vi "multi_column_list_box.vi"() -> ()   [LabVIEW 2023]
uses:
  Values.ctl
panel:
  out "error out":errorcluster
  in  "error in (no error)":errorcluster
  in  "Combo Box":T1
  in  "Multicolumn Listbox":i32[](listbox)=[4] caption="Table"
  in  "stop":bool
  # "Notes:\n    - Hovr the headers of the rows or column to highlisght the entire row or column.\n    - Select the valus present in the drop box to change the vale of the cell."
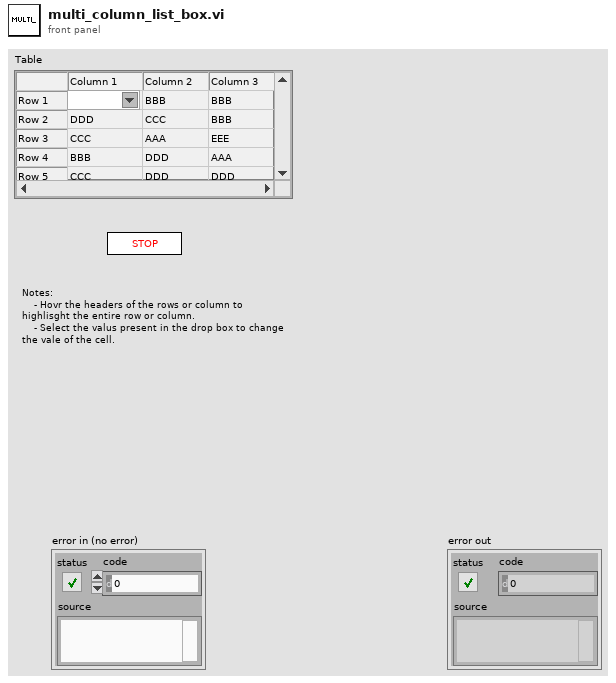
[diagram p1: front panel]
types:
  T1 = typedef "Values.ctl" = string
  T2 = typedef "LVRowAndColumnTypeDef.ctl" = cluster{"Row":i32, "Column":i32}
  T3 = typedef "LVBoundsTypeDef.ctl" = cluster{"Width":u32, "Height":u32}
  T4 = typedef "LVPositionTypeDef.ctl" = cluster{"Left":i32, "Top":i32}
  T5 = typedef "LVPoint32TypeDef.ctl" = cluster{"Horizontal":i32, "Vertical":i32}
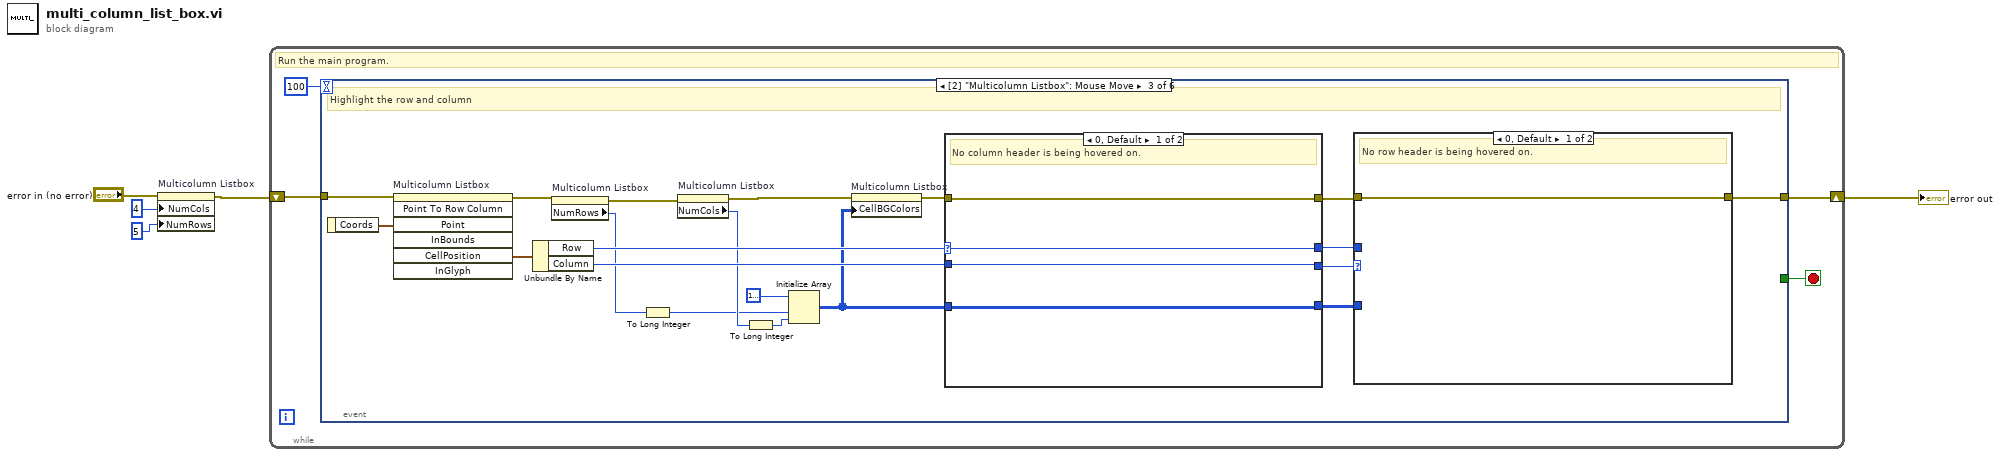
[diagram p0: block diagram]
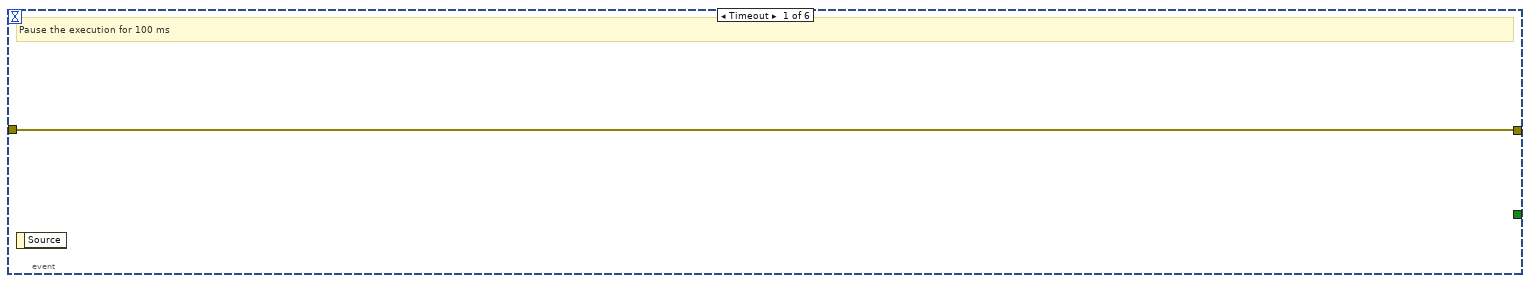
[diagram p2: hidden frame]
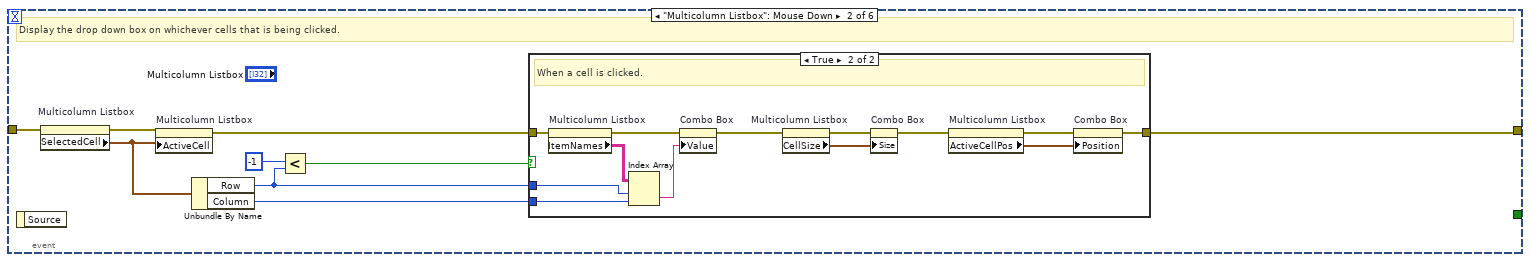
[diagram p3: hidden frame]
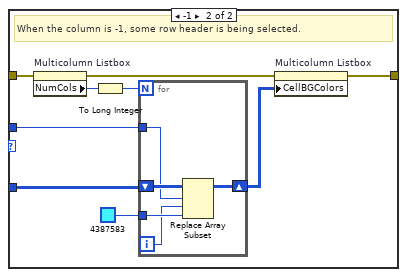
[diagram p5: hidden frame]
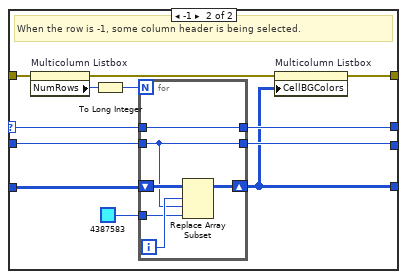
[diagram p6: hidden frame]
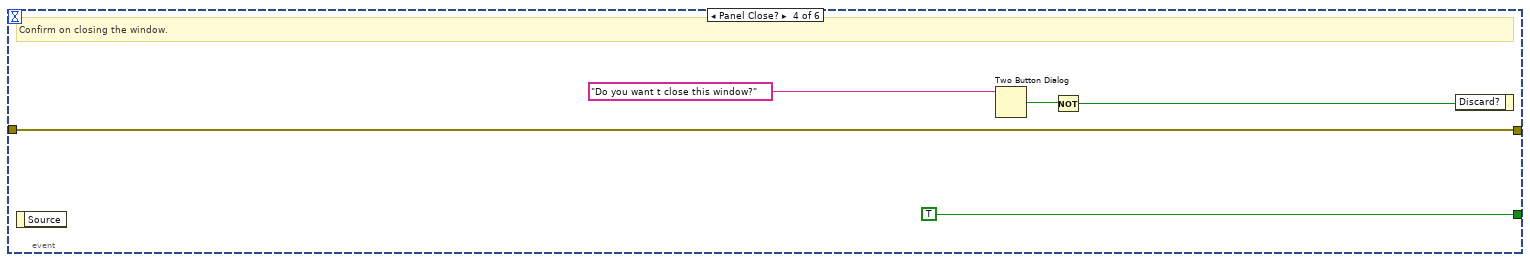
[diagram p7: hidden frame]
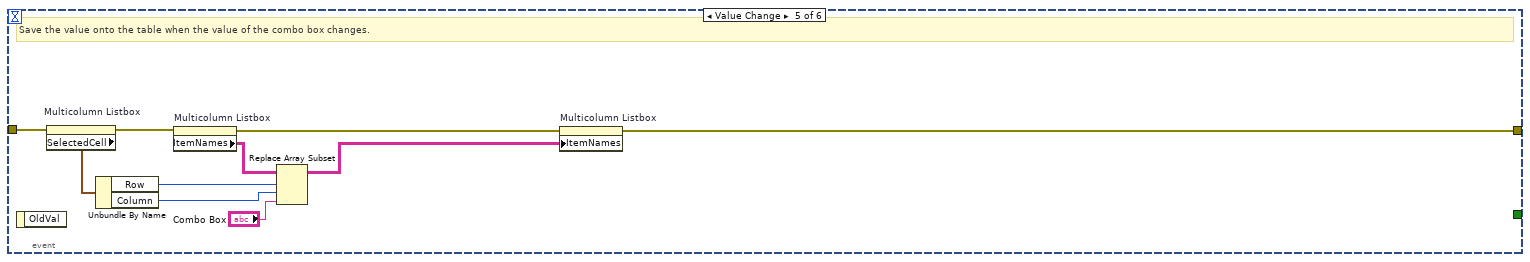
[diagram p8: hidden frame]
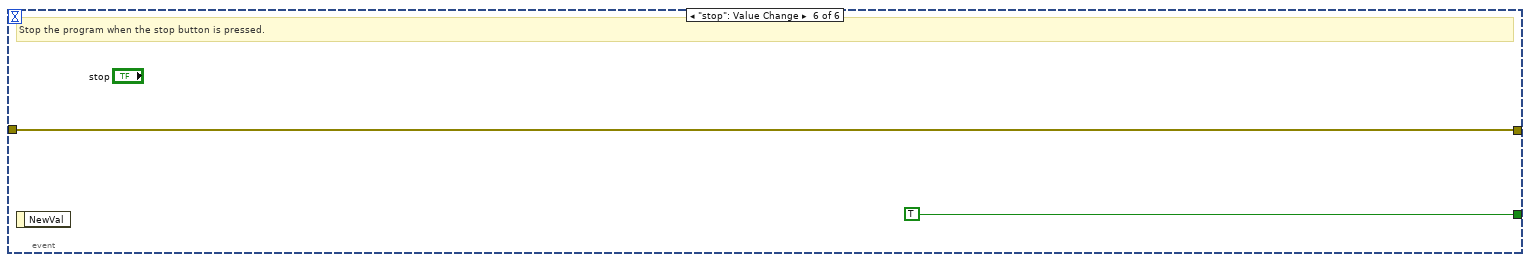
[diagram p9: hidden frame]
diagram:
  n1 = property on="Multicolumn Listbox" class="MCListbox (strict)"(error in="error in (no error)", "NumCols"=u32 4 ("Number of Columns"), "NumRows"=u32 5 ("Number of Rows")) -> (error out=w1:errorcluster)  [unwired: 1 in, 1 out]
  n2 = while {
    shift-right: [w7] -> w5
    shift-left: w1 -> [w6]
    stop <- w9 stop-if-true
    # "Run the main program."
    n3 = event shown="[2] \"Multicolumn Listbox\": Mouse Move" {
      selector: _ -> [_ _ _ _ _ _]
      dyn-events: _ -> [_ _ _ _ _ _]
      timeout: 100 -> [_ _ _ _ _ _]
      tunnel: [_ _ _ TRUE _ TRUE] -> w9
      tunnel: w6 -> [w10 w18 w51 w93 w99 w106]
      tunnel: [w10 w15 w41 w93 w96 w106] -> w7
      event Timeout {
        # "Pause the execution for 100 ms"
        n4 = event-data() -> ()  [unwired: 1 in, 1 out]
      }
      event "Multicolumn Listbox": Mouse Down {
        # "Display the drop down box on whichever cells that is being clicked."
        n5 = event-data() -> ()  [unwired: 1 in, 1 out]
        n6 = property on="Multicolumn Listbox" class="MCListbox (strict)"(error in=w18) -> (error out=w17:errorcluster, "SelectedCell"=w11:T2)  [unwired: 1 in, 1 out]
        n7 = property on="Multicolumn Listbox" class="MCListbox (strict)"(error in=w17, "ActiveCell"=w11) -> (error out=w16:errorcluster)  [unwired: 1 in, 1 out]
        n8 = Unbundle By Name(w11) -> ("Row"=w13:i32, "Column"=w19:i32)
        n9 = Less?(x=-1, y=w13) -> (x < y?=w14:bool)
        n10 = case shown="True" w14 {
          tunnel: w13 -> [_ w32]
          tunnel: w19 -> [_ w31]
          tunnel: w16 -> [w20 w27]
          tunnel: [w20 w21] -> w15
          frame False {
            # "When clicked in the header"
          }
          frame True {
            # "When a cell is clicked."
            n11 = property on="Multicolumn Listbox" class="MCListbox (strict)"(error in=w27) -> (error out=w26:errorcluster, "ItemNames"=w33:string[][])  [unwired: 1 in, 1 out]
            n12 = Index Array(array=w33, index (row)=w32, index (col)=w31) -> (element=w28:string)
            n13 = property on="Combo Box" class="CmbBox (strict)"(error in=w26, "Value"=w28) -> (error out=w25:errorcluster)  [unwired: 1 in, 1 out]
            n14 = property on="Multicolumn Listbox" class="MCListbox (strict)"(error in=w25) -> (error out=w24:errorcluster, "CellSize"=w29:T3)  [unwired: 1 in, 1 out]
            n15 = property on="Combo Box" class="CmbBox (strict)"(error in=w24, "Size"=w29) -> (error out=w23:errorcluster)  [unwired: 1 in, 1 out]
            n16 = property on="Multicolumn Listbox" class="MCListbox (strict)"(error in=w23) -> (error out=w22:errorcluster, "ActiveCellPos"=w30:T4)  [unwired: 1 in, 1 out]
            n17 = property on="Combo Box" class="CmbBox (strict)"(error in=w22, "Position"=w30) -> (error out=w21:errorcluster)  [unwired: 1 in, 1 out]
          }
        }
      }
      event "Multicolumn Listbox": Mouse Move {
        # "Highlight the row and column"
        n18 = event-data() -> ("Coords"=w53:T5)  [unwired: 1 in]
        n19 = invoke on="Multicolumn Listbox" class="MCListbox (strict)" method="Point To Row Column"(error in=w51, "Point"=w53) -> (error out=w36:errorcluster, "CellPosition"=w52:T2)  [unwired: 5 in, 5 out]
        n20 = Unbundle By Name(w52) -> ("Row"=w50:i32, "Column"=w49:i32)
        n21 = property on="Multicolumn Listbox" class="MCListbox (strict)"(error in=w36) -> (error out=w35:errorcluster, "NumRows"=w48:u32)  [unwired: 1 in, 1 out]
        n22 = To Long Integer(number=w48) -> (32bit integer=w46:i32)
        n23 = property on="Multicolumn Listbox" class="MCListbox (strict)"(error in=w35) -> (error out=w34:errorcluster, "NumCols"=w47:u32)  [unwired: 1 in, 1 out]
        n24 = To Long Integer(number=w47) -> (32bit integer=w45:i32)
        n25 = Initialize Array(u32 16777226, w46, w45) -> (w43:u32[][])
        n26 = property on="Multicolumn Listbox" class="MCListbox (strict)"(error in=w34, "CellBGColors"=w43) -> (error out=w42:errorcluster)  [unwired: 1 in, 1 out]
        n27 = case shown="0, Default" w50 {
          selector: w50 -> [w71 w76]
          tunnel: [w72 w78] -> w40
          tunnel: w42 -> [w72 w80]
          tunnel: w49 -> [w70 w83]
          tunnel: w43 -> [w69 w84]
          tunnel: [w71 w75] -> w38
          tunnel: [w70 w74] -> w39
          tunnel: [w69 w73] -> w37
          frame 0, Default {
            # "No column header is being hovered on."
          }
          frame -1 {
            # "When the row is -1, some column header is being selected."
            n28 = property on="Multicolumn Listbox" class="MCListbox (strict)"(error in=w80) -> (error out=w77:errorcluster, "NumRows"=w82:u32)  [unwired: 1 in, 1 out]
            n29 = To Long Integer(number=w82) -> (32bit integer=w81:i32)
            n30 = for {
              N: w81 -> [_]
              tunnel: w83 -> [w85]
              tunnel: u32 4387583 -> [w87]
              shift-right: [w89] -> w73
              shift-left: w84 -> [w90]
              tunnel: w76 -> [w86]
              tunnel: [w86] -> w75
              tunnel: [w85] -> w74
              i -> [w88]
              n31 = Replace Array Subset(array=w90, new element=w87, index (row)=w88, index (col)=w85) -> (w89:u32[][])
            }
            n32 = property on="Multicolumn Listbox" class="MCListbox (strict)"(error in=w77, "CellBGColors"=w73) -> (error out=w78:errorcluster)  [unwired: 1 in, 1 out]
          }
        }
        n33 = case shown="0, Default" w39 {
          tunnel: [w54 w56] -> w41
          tunnel: w40 -> [w54 w58]
          tunnel: w38 -> [_ w62]
          tunnel: w37 -> [_ w63]
          frame 0, Default {
            # "No row header is being hovered on."
          }
          frame -1 {
            # "When the column is -1, some row header is being selected."
            n34 = property on="Multicolumn Listbox" class="MCListbox (strict)"(error in=w58) -> (error out=w55:errorcluster, "NumCols"=w60:u32)  [unwired: 1 in, 1 out]
            n35 = To Long Integer(number=w60) -> (32bit integer=w59:i32)
            n36 = for {
              N: w59 -> [_]
              tunnel: w62 -> [w65]
              tunnel: u32 4387583 -> [w66]
              shift-right: [w67] -> w61
              shift-left: w63 -> [w68]
              i -> [w64]
              n37 = Replace Array Subset(array=w68, new element=w66, index (row)=w65, index (col)=w64) -> (w67:u32[][])
            }
            n38 = property on="Multicolumn Listbox" class="MCListbox (strict)"(error in=w55, "CellBGColors"=w61) -> (error out=w56:errorcluster)  [unwired: 1 in, 1 out]
          }
        }
      }
      event Panel Close? {
        # "Confirm on closing the window."
        n39 = event-data() -> ()  [unwired: 1 in, 1 out]
        n40 = Two Button Dialog(message="Do you want t close this window?") -> (T button?=w91:bool)  [unwired: 2 in]
        n41 = Not(x=w91) -> (.not. x?=w92:bool)
        n42 = event-data("Discard?"=w92) -> ()  [unwired: 1 in, 1 out]
      }
      event Value Change {
        # "Save the value onto the table when the value of the combo box changes."
        n43 = event-data() -> ()  [unwired: 1 in, 1 out]
        n44 = property on="Multicolumn Listbox" class="MCListbox (strict)"(error in=w99) -> (error out=w98:errorcluster, "SelectedCell"=w105:T2)  [unwired: 1 in, 1 out]
        n45 = Unbundle By Name(w105) -> ("Row"=w103:i32, "Column"=w102:i32)
        n46 = property on="Multicolumn Listbox" class="MCListbox (strict)"(error in=w98) -> (error out=w97:errorcluster, "ItemNames"=w104:string[][])  [unwired: 1 in, 1 out]
        n47 = Replace Array Subset(array=w104, new element="Combo Box", index (row)=w103, index (col)=w102) -> (w101:string[][])
        n48 = property on="Multicolumn Listbox" class="MCListbox (strict)"(error in=w97, "ItemNames"=w101) -> (error out=w96:errorcluster)  [unwired: 1 in, 1 out]
      }
      event "stop": Value Change {
        # "Stop the program when the stop button is pressed."
        n49 = event-data() -> ()  [unwired: 1 in, 1 out]
      }
    }
  }
  "error out" <- w5
